vi "Save sequence into multiple images.vi"(3 "Header file data":T1 {"Pixel depth" items=["8 bits", "16 bits", "Float", "Complex", "RGB", "HSL"]; "time of 1st frame, \nsec since 1/1/04" format="%.2f"}, 4 "Acqisition files refnums":refnum<file>[](array[refnum]), 5 "starting frame number to save":u32, 6 "File Format":string="TIFF", 7 "error in":errorcluster, 8 "Number of frames to save":u32, 9 "AOI List":u16[][](array[numeric]), 10 "Directory path":path) -> (0 "error out":errorcluster)   [LabVIEW 2016]
doc: "Save sequence into multiple images in a directory.\n\nINPUTS:\nDirectory name (sequence name with path). If left empty, the program will prompt for name.\nSequence of images.\nFile format (AIPD as default)"
uses:
  Header file data.ctl
  Seq file v 1/Offset table.ctl
  Seq file v 1/Offset.ctl
  Seq file v 1/file number.ctl
panel:
  in  "Quit":bool
  out "Frame number":u32
  out "AOI number":i32
  out "File":path
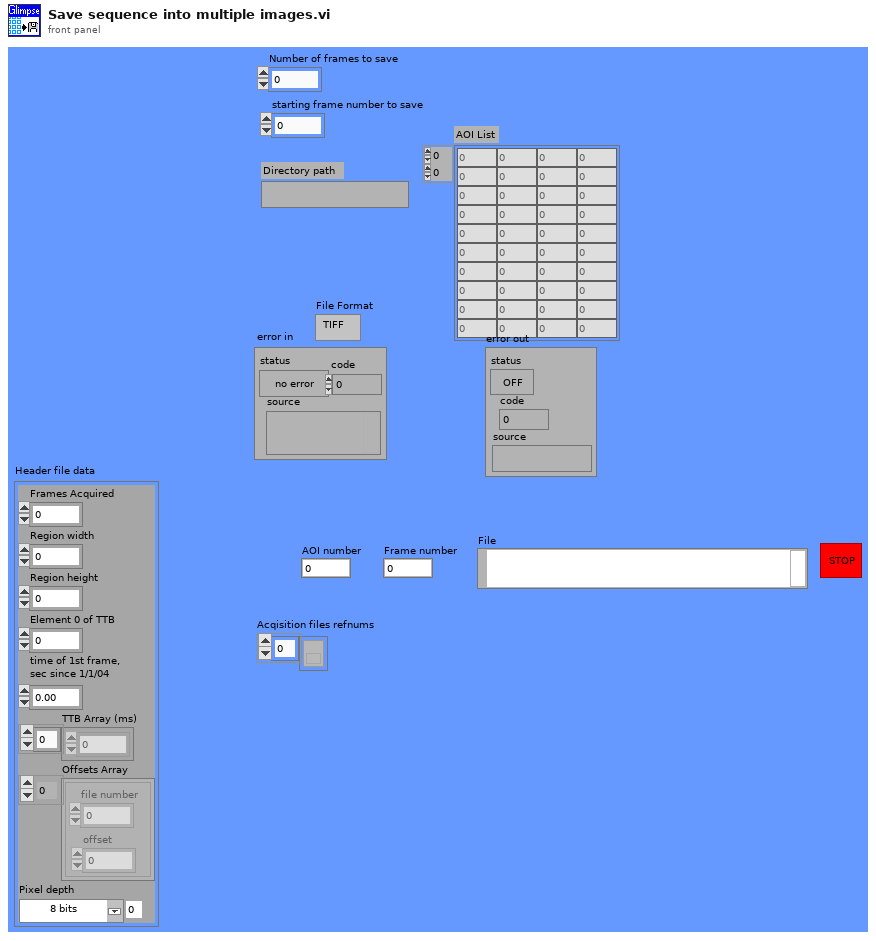
[diagram p1: front panel]
types:
  T1 = typedef "Header file data.ctl" = cluster{"Frames Acquired":u32, "Region width":i32, "Region height":i32, "Element 0 of TTB":u32, "time of 1st frame, \nsec since 1/1/04":dbl, "TTB Array (ms)":u32[], "Offsets Array":T2, "Pixel depth":u32}
  T2 = typedef "Offset table.ctl" = cluster{"offset":T3, "file number":T4}[]
  T3 = typedef "Offset.ctl" = i32
  T4 = typedef "file number.ctl" = u8
  T5 = cluster{"Rows Per Strip":i32, "Photometric":i32, "Compression Type":i32}
  T6 = enum32{"existing file", "new file", "new or existing file", "existing dir", "new dir", "new or existing dir", "existing file (use LLBs)", "new file (use LLBs)", "new or existing file (use LLBs)", "new or existing file or directory (use LLBs)"}
  T7 = typedef "IMAQ Image.ctl" = refnum<image>
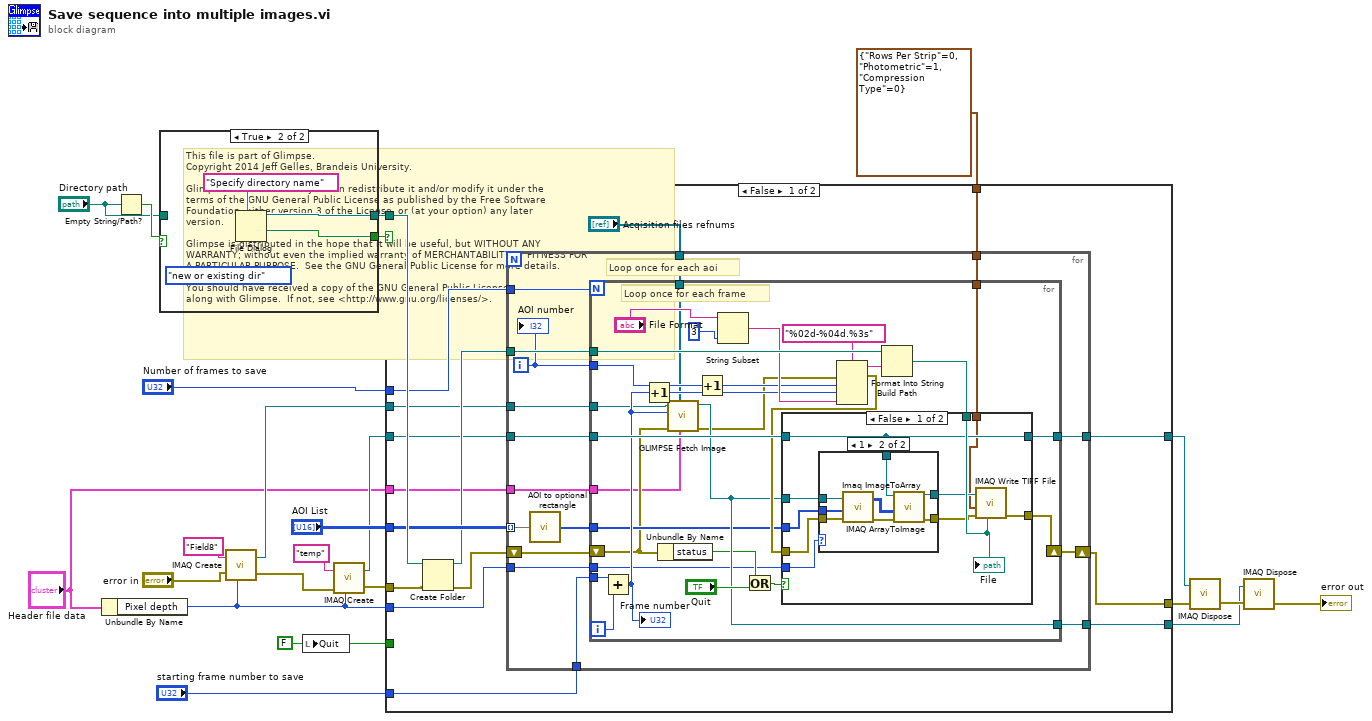
[diagram p0: block diagram]
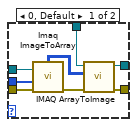
[diagram p2: hidden frame]
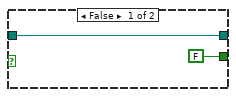
[diagram p5: hidden frame]
diagram:
  w18 = FALSE ("Quit")
  # "This file is part of Glimpse. \nCopyright 2014 Jeff Gelles, Brandeis University.    \n\nGlimpse is free software: you can redistribute it and/or modify it under the \nterms of the GNU General Public License as published by the Free Software \nFoundation, either version 3 of the License, or (at your option) any later \nversion.\n\nGlimpse is distributed in the hope that it will be useful, but WITHOUT ANY \nWARRANTY; without even the implied warranty of MERCHANTABILITY or FITNESS FOR \nA PARTICULAR PURPOSE.  See the GNU General Public License for more details.\n\nYou should have received a copy of the GNU General Public License\nalong with Glimpse.  If not, see <http://www.gnu.org/licenses/>."
  n1 = Unbundle By Name("Header file data") -> ("Pixel depth"=w2:u32)
  n2 = Empty String/Path?(string/path="Directory path") -> (empty?=w23:bool)
  n3 = case shown="True" w23 {
    tunnel: [w25 w28] -> w21
    tunnel: "Directory path" -> [w25 _]
    tunnel: [FALSE ("cancelled") w26] -> w20
    frame False {
    }
    frame True {
      (unwired) T6."new or existing dir" ("select mode (2)")
      n4 = File Dialog(7:"Specify directory name" ("prompt")) -> (1:w26:bool, 3:w28:path)  [unwired: 1 in, 7 out]
    }
  }
  n5 = call "IMAQ Create"("Image Name"="Field8", "Image Type"=w2, "error in (no error)"="error in") -> ("New Image"=w11:T7, "error out"=w9:errorcluster)  [unwired: 1 in, 1 out]
  n6 = local write "Quit"(w18) -> ()
  n7 = call "IMAQ Create"("Image Name"="temp", "Image Type"=w2, "error in (no error)"=w9) -> ("New Image"=w15:T7, "error out"=w16:errorcluster)  [unwired: 1 in, 1 out]
  n8 = case shown="False" w20 {
    tunnel: w21 -> [w44 _]
    tunnel: "AOI List" -> [w43 _]
    tunnel: w16 -> [w40 w120]
    tunnel: [w42 w120] -> w14
    tunnel: w18 -> [_ _]
    tunnel: w15 -> [w38 w119]
    tunnel: [w37 w119] -> w13
    tunnel: "Number of frames to save" -> [w36 _]
    tunnel: w11 -> [w35 w118]
    tunnel: [w34 w118] -> w7
    tunnel: "starting frame number to save" -> [w33 _]
    tunnel: "Header file data" -> [w31 _]
    tunnel: w2 -> [w30 _]
    tunnel: T5 {"Rows Per Strip"=0, "Photometric"=1, "Compression Type"=0} ("TIFF Options") -> [w29 _]
    frame False {
      n9 = Create Folder(path (use dialog)=w44, error in=w40) -> (created path=w41:path, error out=w39:errorcluster)  [unwired: 2 out]
      n10 = for {
        tunnel: w43 -> [w48] mode=indexing
        shift-right: [w59] -> w42
        shift-left: w39 -> [w60]
        tunnel: w41 -> [w58]
        tunnel: w38 -> [w57]
        tunnel: [w56] -> w37
        tunnel: w36 -> [w54]
        tunnel: w35 -> [w53]
        tunnel: [w52] -> w34
        tunnel: w33 -> [w51]
        tunnel: "Acqisition files refnums" -> [w50]
        tunnel: w31 -> [w47]
        tunnel: w30 -> [w46]
        tunnel: w29 -> [w45]
        i -> [w55]
        # "Loop once for each aoi"
        # "Loop once for each aoi"
        n11 = call "AOI to optional rectangle.vi"("x1, y1, x2, y2 with origin (0, 0)"=w48) -> ("x1, y1, x2+1, y2+1 with origin (0, 0)"=w49:u16[])  [unwired: 4 out]
        n12 = for {
          N: w54 -> [_]
          tunnel: w49 -> [w68]
          shift-right: [w85] -> w59
          shift-left: w60 -> [w66]
          tunnel: w58 -> [w88]
          tunnel: w57 -> [w83]
          tunnel: [w82] -> w56
          tunnel: w55 -> [w81]
          tunnel: w53 -> [w73]
          tunnel: [w70] -> w52
          tunnel: w51 -> [w71]
          tunnel: w50 -> [w69]
          tunnel: w47 -> [w63]
          tunnel: w46 -> [w62]
          tunnel: w45 -> [w61]
          i -> [w72]
          # "Loop once for each frame"
          # "Loop once for each frame"
          n13 = Add(x=w71, y=w72) -> (x+y=w74:u32)
          "Frame number" <- w74
          n14 = Increment(x=w74) -> (x+1=w76:u32)
          n15 = Unbundle By Name(w66) -> ("status"=w64:bool)
          n16 = call "GLIMPSE Fetch Image.vi"("Header file data"=w63, "Acqisition files refnums"=w69, "error in"=w66, "Logical Frame Number\n(starting with zero)"=w74, "Image In"=w73) -> ("error out"=w67:errorcluster, "Image Out"=w70:T7)  [unwired: 2 in, 3 out]
          n17 = Increment(x=w81) -> (x+1=w75:i32)
          n18 = String Subset(string="File Format", length (rest)=3 ("length")) -> (substring=w77:string)  [unwired: 1 out]
          n19 = Or(x=w64, y="Quit") -> (x .or. y?=w65:bool)
          n20 = Format Into String(format string="%02d-%04d.%3s" ("Format String"), error in=w67, w75, w76, w77) -> (resulting string=w79:string, error out=w80:errorcluster)  [unwired: 1 in]
          n21 = Build Path(base path=w88, name or relative path=w79) -> (appended path=w89:path)
          n22 = case shown="False" w65 {
            tunnel: w89 -> [w99 _]
            tunnel: w68 -> [w98 _]
            tunnel: w70 -> [w97 _]
            tunnel: w80 -> [w95 w117]
            tunnel: [w93 w117] -> w85
            tunnel: w83 -> [w92 w116]
            tunnel: [w92 w116] -> w82
            tunnel: w62 -> [w91 _]
            tunnel: w61 -> [w90 _]
            frame False {
              n23 = case shown="1" w91 {
                tunnel: w98 -> [w107 w111]
                tunnel: w97 -> [w106 w113]
                tunnel: [w104 w110] -> w96
                tunnel: w95 -> [w102 w112]
                tunnel: [w101 w109] -> w94
                tunnel: w92 -> [w100 w114]
                frame 0, Default {
                  n24 = call "Imaq ImageToArray"("error in (no error)"=w102, "Optional Rectangle"=w107, "Image"=w106) -> ("error out"=w103:errorcluster, "Image Pixels (U8)"=w105:u8[][])  [unwired: 4 out]
                  n25 = call "IMAQ ArrayToImage"("error in (no error)"=w103, "Image Pixels (U8)"=w105, "Image"=w100) -> ("error out"=w101:errorcluster, "Image Out"=w104:T7)  [unwired: 3 in, 4 out]
                }
                frame 1 {
                  n26 = call "Imaq ImageToArray"("error in (no error)"=w112, "Optional Rectangle"=w111, "Image"=w113) -> ("error out"=w115:errorcluster, "Image Pixels (I16)"=w108:i16[][])  [unwired: 4 out]
                  n27 = call "IMAQ ArrayToImage"("error in (no error)"=w115, "Image Pixels (I16)"=w108, "Image"=w114) -> ("error out"=w109:errorcluster, "Image Out"=w110:T7)  [unwired: 3 in, 4 out]
                }
              }
              n28 = call "IMAQ Write TIFF File"("error in (no error)"=w94, "TIFF Options"=w90, "File Path"=w99, "Image"=w96) -> ("error out"=w93:errorcluster)  [unwired: 1 in, 3 out]
              "File" <- w99
            }
            frame True {
            }
          }
        }
        "AOI number" <- w55
      }
    }
    frame True {
    }
  }
  n29 = call "IMAQ Dispose"("Image"=w13, "error in (no error)"=w14) -> ("error out"=w8:errorcluster)  [unwired: 1 in, 3 out]
  n30 = call "IMAQ Dispose"("Image"=w7, "error in (no error)"=w8) -> ("error out"=→"error out":errorcluster)  [unwired: 1 in, 3 out]
